vi "draw current_tour on chessboard.vi"(11 "current_tour":T1[](array[typedef])) -> (3 "Chess board":bool[][](array[boolean]))   [LabVIEW 2020, in "main.lvlib"]
uses:
  main.lvlib
  core/core_data/chessboard_index.ctl
  core/core_data/core_data.lvlib
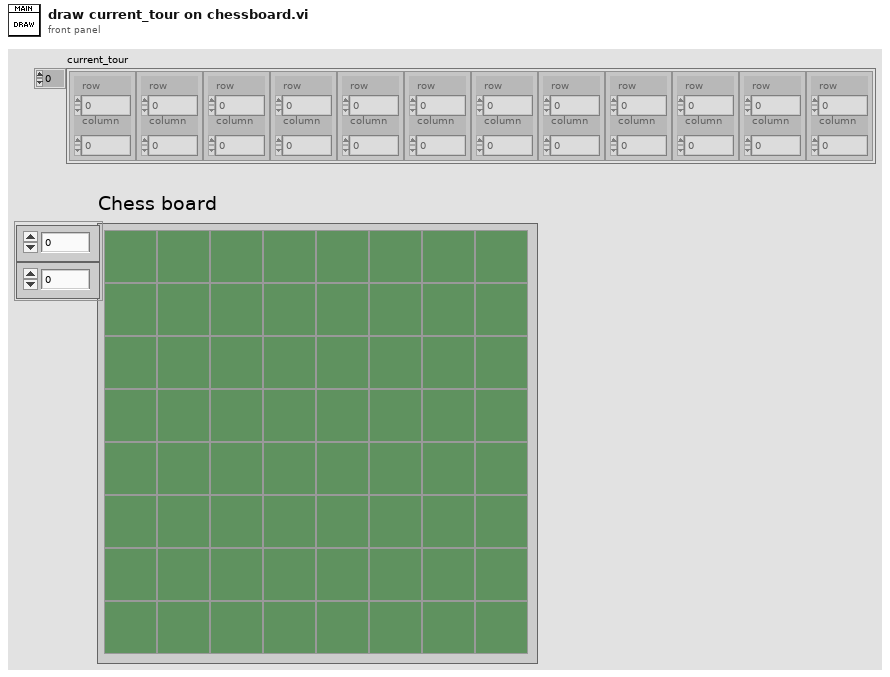
[diagram p1: front panel]
types:
  T1 = typedef "core.lvlib/core_data.lvlib/chessboard_index.ctl" = cluster{"row":u8, "column":u8}
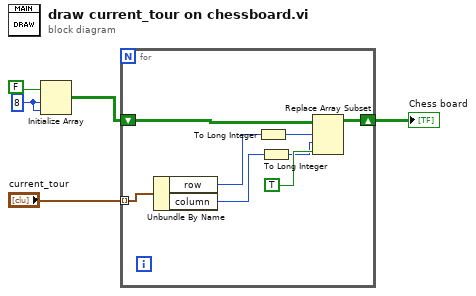
[diagram p0: block diagram]
diagram:
  w3 = 8 ("dimension size")
  n1 = Initialize Array(FALSE, w3, w3) -> (w4:bool[][])
  n2 = for {
    shift-right: [w12] -> w1
    shift-left: w4 -> [w13]
    tunnel: "current_tour" -> [w10] mode=indexing
    n3 = Unbundle By Name(w10) -> ("row"=w9:u8, "column"=w8:u8)
    n4 = To Long Integer(number=w9) -> (32bit integer=w7:i32)
    n5 = To Long Integer(number=w8) -> (32bit integer=w6:i32)
    n6 = Replace Array Subset(array=w13, new element=TRUE ("new element/subarray"), index (row)=w7, index (col)=w6) -> (w12:bool[][])
  }
  "Chess board" <- w1
